vi "3.6-Cerebellum.vi"() -> ()   [LabVIEW 2010]
uses:
  4-High Neurons/4.1.2-Act Neuron TD.ctl
  3.0 Flow Control/3.0 List of Loops.ctl
  3.0-Global.vi
  <vilib>/robotics/Obstacle Avoidance/Advanced Vector Field Histogram/NI_Robotics_Vector Field Histogram.lvlib
panel:
  out "Dont Run!":bool
  out "Input Act Neurons":T1
  in  "heading (Degrees)":T2
  out "chosen heading (rad)":dbl
  out "Heartbeat":bool
  out "error out":errorcluster
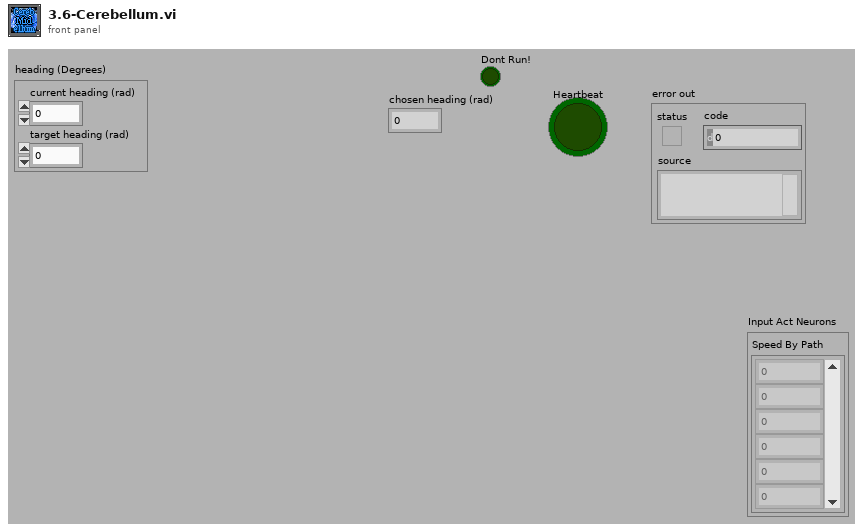
[diagram p1: front panel]
types:
  T1 = typedef "4.1.2-Act Neuron TD.ctl" = cluster{"Speed By Path":sgl[]}
  T2 = cluster{"current heading (rad)":dbl, "target heading (rad)":dbl}
  T3 = typedef "3.0 List of Loops.ctl" = enum16{"3.0 State Update", "3.0 GUI", "3.1 Act", "3.1 4.7.1 Act UDP", "3.1 Joystick", "3.2 Where", "3.2 4.7.2 Where UDP", "3.3 What", "3.3 4.7.3 What UDP", "3.4 How", "3.4 4.7.4 How UDP", "3.5 Limbic", "3.8 TCP", "3.6 Cerebellum", "3.8 TCP Act"}
  T4 = enum16{"Set Joystick", "Read Joystick", "Set Forebrain", "Read Forebrain", "Set Limbic", "Read Limbic", "Set Cerebellum", "Read Cerebellum", "Set Arbitrated", "Read Arbitrated", "Set LIDAR", "Read LIDAR"}
  T5 = cluster{"inner threshold distance":dbl, "outer threshold distance":dbl}
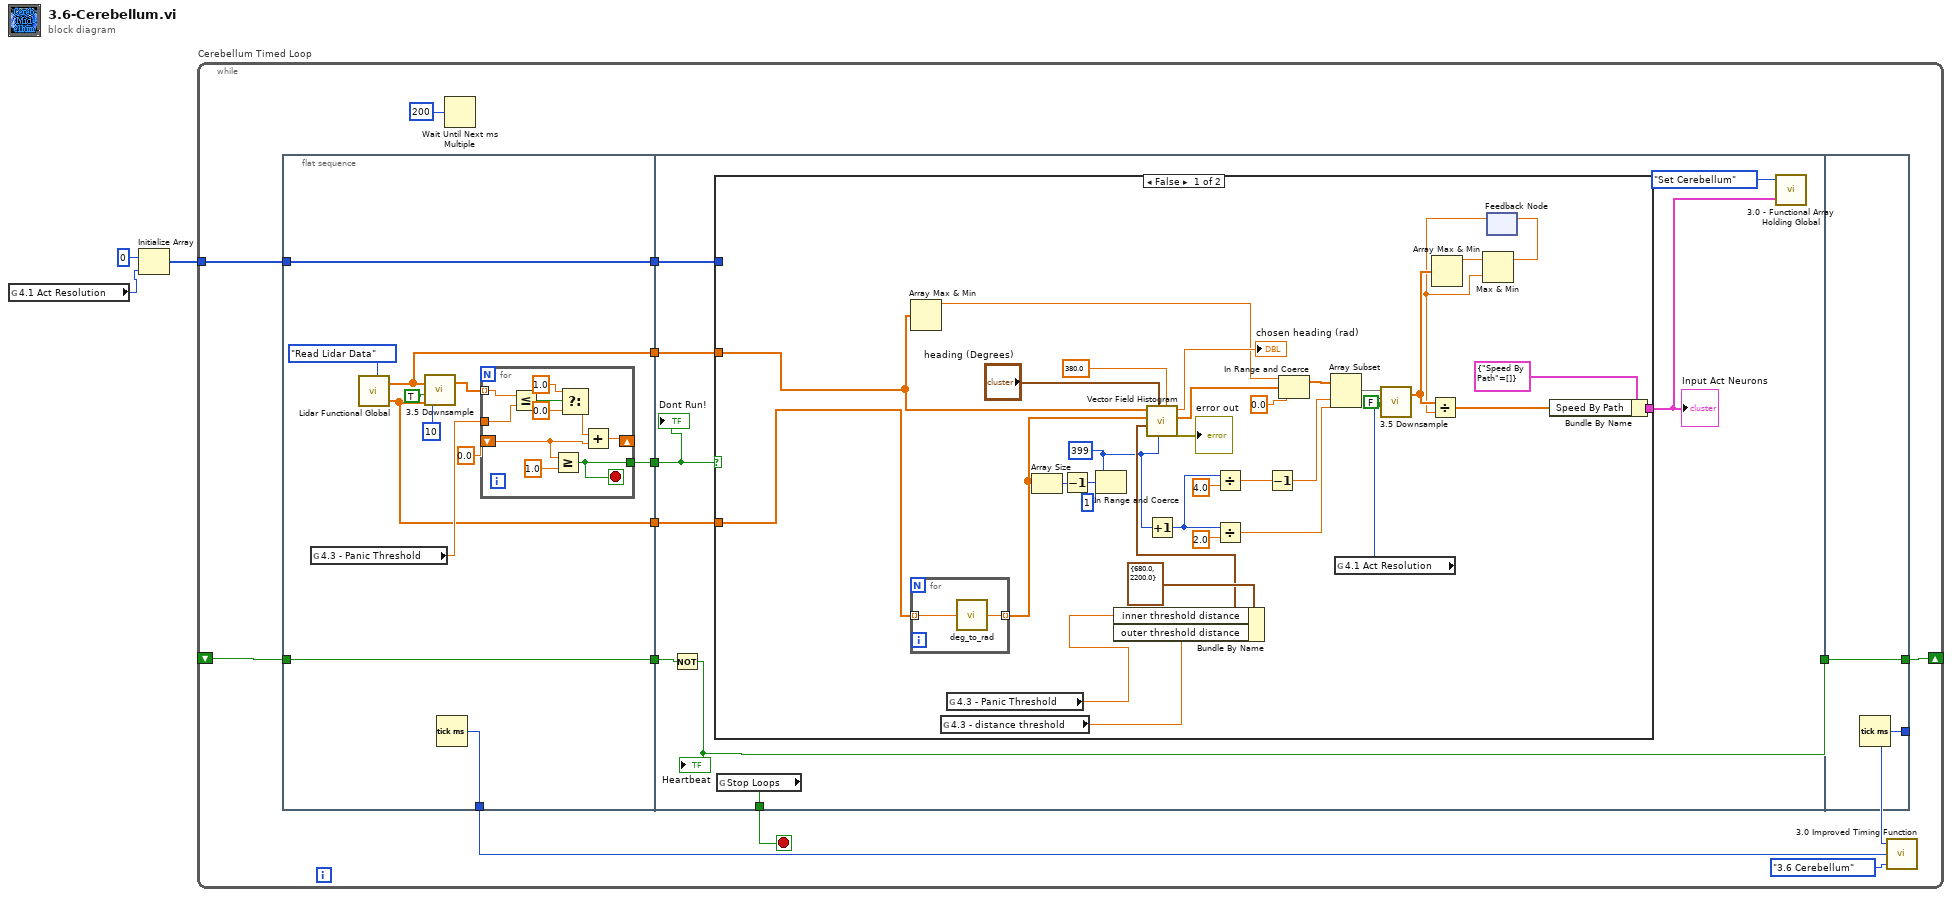
[diagram p0: block diagram]
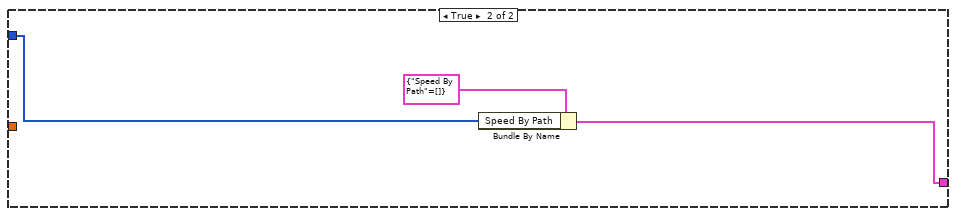
[diagram p2: hidden frame]
diagram:
  n1 = global read "3.0-Global.vi" "4.1 Act Resolution"() -> (w3:u32)
  n2 = Initialize Array(u32 0 ("element"), w3) -> (w1:u32[])
  n3 = while "Cerebellum Timed Loop" {
    shift-right: [w16] -> _
    shift-left: _ -> [w17]
    tunnel: w1 -> [w6]
    stop <- w4 stop-if-true
    n4 = flat-sequence {
      tunnel: w17 -> [w29]
      tunnel: [w29] -> w15
      tunnel: [w28] -> w12
      tunnel: [w24] -> w9
      tunnel: [w18] -> w8
      tunnel: [w21] -> w7
      tunnel: w6 -> [w20]
      tunnel: [w20] -> w5
      tunnel: w15 -> [w48]
      tunnel: [w41] -> w14
      tunnel: w9 -> [w46]
      tunnel: w8 -> [w45]
      tunnel: w7 -> [w40]
      tunnel: w5 -> [w43]
      tunnel: [w42] -> w4
      tunnel: [w90] -> w16
      tunnel: w14 -> [w90]
      tunnel: [w89] -> w13
      frame #0 {
        n5 = global read "3.0-Global.vi" "4.3 - Panic Threshold"() -> (w19:dbl)
        n6 = call "Lidar Functional Global.vi"("Lidar Action"=enum16{"Set Lidar Data", "Read Lidar Data"}."Read Lidar Data") -> ("Lidar Angle Data Out (Degrees)"=w18:sgl[], "Lidar Magnitude Data Out (mm)"=w24:sgl[])  [unwired: 2 in]
        n7 = call "3.5 Downsample.vi"("Corresponding Input Array For Minimum"=w18, "Minimum?"=TRUE, "Numeric"=10, "Input Array"=w24) -> ("Output Array"=w23:sgl[])  [unwired: 1 out]
        n8 = Tick Count (ms)() -> (millisecond timer value=w28:u32)
        n9 = for {
          shift-right: [w33] -> _
          shift-left: 0.0 -> [w32]
          tunnel: w23 -> [w39] mode=indexing
          tunnel: w19 -> [w38]
          tunnel: [w30] -> w21
          stop <- w30 stop-if-true
          n10 = Less Or Equal?(x=w39, y=w38) -> (x <= y?=w37:bool)
          n11 = Greater Or Equal?(x=w32, y=1.0) -> (x >= y?=w30:bool)
          n12 = Select(t=1.0, s=w37, f=0.0) -> (s? t:f=w34:dbl)
          n13 = Add(x=w34, y=w32) -> (x+y=w33:dbl)
        }
      }
      frame #1 {
        n14 = Not(x=w48) -> (.not. x?=w41:bool)
        "Heartbeat" <- w41
        n15 = case shown="False" w40 {
          tunnel: [w73 w86] -> w47
          tunnel: w46 -> [w50 _]
          tunnel: w45 -> [w49 _]
          tunnel: w43 -> [_ w87]
          frame False {
            w52 = 399 ("# bins")
            n16 = Array Max & Min(array=w50) -> (max value=w71:sgl)  [unwired: 3 out]
            n17 = for {
              tunnel: w49 -> [w85] mode=indexing
              tunnel: [w84] -> w56 mode=indexing
              n18 = call "deg_to_rad.vi"("Degrees"=w85) -> ("Radians"=w84:dbl)
            }
            n19 = global read "3.0-Global.vi" "4.3 - distance threshold"() -> (w82:dbl)
            n20 = global read "3.0-Global.vi" "4.3 - Panic Threshold"() -> (w83:dbl)
            n21 = Array Size(array=w56) -> (size(s)=w55:i32)
            n22 = Decrement(x=w55) -> (x-1=w53:i32)
            n23 = In Range and Coerce(upper limit=w52, x=w53, lower limit=1) -> ()  [unwired: 2 out]
            n24 = Bundle By Name(cluster=T5 {"inner threshold distance"=680.0, "outer threshold distance"=2200.0} ("thresholds"), "inner threshold distance"=w83, "outer threshold distance"=w82) -> (w57:T5)
            n25 = call <vilib>:"Vector Field Histogram.vi"("obstacle clearance distance"=380.0, "# bins"=w52, "heading"="heading (Degrees)", "thresholds"=w57, "direction angles (rad)"=w56, "distances"=w50) -> ("error out"=→"error out":errorcluster, "histogram"=w60:dbl[], "chosen heading (rad)"=→"chosen heading (rad)":dbl)  [unwired: 2 in, 1 out]
            n26 = Increment(x=w52) -> (x+1=w61:i32)
            n27 = Divide(x=w61, y=4.0) -> (x/y=w66:dbl)
            n28 = Divide(x=w61, y=2.0) -> (x/y=w63:dbl)
            n29 = Decrement(x=w66) -> (x-1=w65:dbl)
            n30 = In Range and Coerce(upper limit=w71, x=w60, lower limit=0.0 ("obstacle clearance distance")) -> (coerced(x)=w59:dbl[])  [unwired: 1 out]
            n31 = Array Subset(array=w59, index=w65, length=w63) -> (w62:dbl[])
            n32 = global read "3.0-Global.vi" "4.1 Act Resolution"() -> (w77:u32)
            n33 = call "3.5 Downsample.vi"("Minimum?"=FALSE, "Numeric"=w77, "Input Array"=w62) -> ("Output Array"=w72:sgl[])  [unwired: 1 in, 1 out]
            n34 = Array Max & Min(array=w72) -> (max value=w79:sgl)  [unwired: 3 out]
            n35 = feedback #1() -> (w69:sgl)  [unwired: 1 in]
            n36 = Divide(x=w72, y=w69) -> (x/y=w68:sgl[])
            n37 = Max & Min(x=w79, y=w69) -> (max(x,y)=w78:sgl)  [unwired: 1 out]
            n38 = feedback-in #1(w78) -> ()
            n39 = Bundle By Name(cluster=T1 {"Speed By Path"=[]} ("Input Act Neurons"), "Speed By Path"=w68) -> (w73:T1)
          }
          frame True {
            n40 = Bundle By Name(cluster=T1 {"Speed By Path"=[]} ("Input Act Neurons"), "Speed By Path"=w87) -> (w86:T1)
          }
        }
        "Input Act Neurons" <- w47
        n41 = global read "3.0-Global.vi" "Stop Loops"() -> (w42:bool)
        n42 = call "3.0 - Functional Array Holding Global.vi"("Input Act Neurons"=w47, "Mode"=T4."Set Cerebellum") -> ()  [unwired: 1 out]
        "Dont Run!" <- w40
      }
      frame #2 {
        n43 = Tick Count (ms)() -> (millisecond timer value=w89:u32)
      }
    }
    n44 = Wait Until Next ms Multiple(millisecond multiple=u32 200) -> ()  [unwired: 1 out]
    n45 = call "3.0 Improved Timing Function.vi"("Loop"=3.0_List_of_Loops."3.6 Cerebellum", "Start"=w12, "End"=w13) -> ()  [unwired: 1 in]
  }
